vi "Tag Names.vi"(11 "State in":T2={"State"=enum."Idle", "Start Time"=timestamp(0 s since 1904-01-01), "Configuration"={"Cycle Period"=0.0, "Ismatech"={"VISA resource name"="", "Simulated?"=FALSE, "Pump Number"=1.0, "Reverse?"=FALSE}, "Masterflex"={"VISA resource name"="", "Simulated?"=FALSE, "Pump Number"=1.0, "Reverse?"=FALSE}, "Mettler"={"VISA resource name"="", "Simulated?"=FALSE}, "Bronkhorst M13 Flow Meter"={"VISA resource name"="", "Simulated?"=FALSE}, "PID 2 Parameters"={"Input Device"=enum."Bronkhorst M13", "Output Device"=enum."Ismatec ISM 831C", "Setpoint"=0.0, "PID gains"={"proportional gain (Kc)"=1.0, "integral time (Ti, min)"=0.01, "derivative time (Td, min)"=0.0}}, "Manual Entry"=0.0, "Auto?"=TRUE, "output range"={"output high"=100.0, "output low"=0.0}, "Bronkhorst M14"={"VISA resource name"="", "Simulated?"=FALSE}, "Tacmina Settings"={"Analog DAQ Task"="", "Digital DAQ Task"=""}, "KNF SIMDOS Settings"={"VISA resource name"="", "Simulated?"=TRUE}, "ASIA Pump C"={"ASIA Pump #"=0, "channel"=0, "Simulated"=FALSE}, "VICI Settings"={"VISA resource name"="", "Simulated?"=FALSE, "Pump Letter"="", "Reverse?"=FALSE}, "FLOM Settings"={"VISA resource name"="", "Simulated?"=TRUE, "Pump Number"=0.0}, "SSI PR Settings"={"VISA resource name"="", "Simulated?"=FALSE}}, "Current Time"=timestamp(0 s since 1904-01-01), "PID 1 Parameters"={"Setpoint"=0.0, "PID gains"={"proportional gain (Kc)"=1.0, "integral time (Ti, min)"=0.01, "derivative time (Td, min)"=0.0}}, "First Iteration"=FALSE, "Data"={"Flowmeter Output"=0.0, "Density"=0.0, "FL Temp"=0.0, "Scale Output (g)"=0.0, "Scale Rate of Change (g/min)"=0.0, "PID 1 Output"=0.0, "PID 2 Process Variable"=0.0, "PID 2 output"=0.0, "Pump Flow"=0.0, "Pump Pressure"=0.0}, "Process Name"="", "Pump On?"=enum."Off", "Input Error"=FALSE, "Output Error"=FALSE, "Log Started"=FALSE, "Current Setpoint"=0.0} {"PID 1 Parameters"."PID gains"."derivative time (Td, min)" format="%.3f"; "PID 1 Parameters"."PID gains"."integral time (Ti, min)" format="%.3f"; "PID 1 Parameters"."PID gains"."proportional gain (Kc)" format="%.3f"; "Configuration"."output range"."output low" min=0.0 max=100.0 format="%.2f"; "Configuration"."output range"."output high" format="%.2f"; "Configuration"."PID 2 Parameters"."PID gains"."derivative time (Td, min)" format="%.3f"; "Configuration"."PID 2 Parameters"."PID gains"."integral time (Ti, min)" format="%.3f"; "Configuration"."PID 2 Parameters"."PID gains"."proportional gain (Kc)" format="%.3f"; "Configuration"."ASIA Pump C"."channel" min=0 max=1 step=1; "Configuration"."Ismatech"."Pump Number" min=1.0 max=20.0 step=1.0; "Configuration"."Masterflex"."Pump Number" min=1.0 max=20.0 step=1.0}) -> (0 "All  Flow Meter Tags":string[](array[string]), 1 "All  Scale Tags":string[](array[string]), 3 "Feed Module Tag Names":T1, 4 "All Boolean Tags":string[](array[string]), 5 "All  Numeric Tags":string[](array[string]))   [LabVIEW 2018, in "Feed Module.lvlib" / "Feed Module Engine.lvlib"]
uses:
  Feed Module Engine.lvlib
  State Cluster.ctl
  State Enum.ctl
  Feed Module/Controls/Feed Module Settings Cluster.ctl
  Ismatec ISM 831C/Controls/Ismatech Settings Cluster.ctl
  Masterflex 7550-30/Controls/Settings Cluster.ctl
  Mettler Toledo/Controls/Settings Cluster.ctl
  Bronkhorst M13 Flow Meter/Settings Cluster.ctl
  PID 2 Parameters Cluster.ctl
  PID Input Enum.ctl
  PID 2 Output Enum.ctl
  Tacmina QI/Tacmina QI DAQ Setting.ctl
  KNF Pump/Settings Cluster plus SIMDOS.ctl
  ASIA Pump/Pump Settings.ctl
  VICI M50 Party Mode/Settings Cluster.ctl
  FLOM Pump/Settings Cluster.ctl
  SSI PR Class/SSI PR Settings Cluster.ctl
  PID 1 Parameters Cluster.ctl
  Feed Module/Controls/Feed Module Tag Names Cluster.ctl
  Feed Module/Feed Module.lvlib
  Ismatec ISM 831C/Ismatec ISM 831C.lvlib
  Masterflex 7550-30/Masterflex 7550-30.lvlib
  Mettler Toledo/Mettler Toledo.lvlib
  Bronkhorst M13 Flow Meter/Bronkhorst M13 Flow Meter.lvlib
  Tacmina QI/Tacmina QI.lvlib
  KNF Pump/KNF SIMDOS.lvlib
  ASIA Pump.lvlib
  VICI M50 Party Mode/VICI M6 M50 Party Mode.lvlib
  FLOM Pump/FLOM Pump.lvlib
  SSI PR Class/SSI PR Pump.lvlib
panel:
  out "Pump Flow Tag":string
  out "PID 2 Out Tag":string
  out "Scale Tag":string
  # "Output Instruments"
  # "Input Instruments"
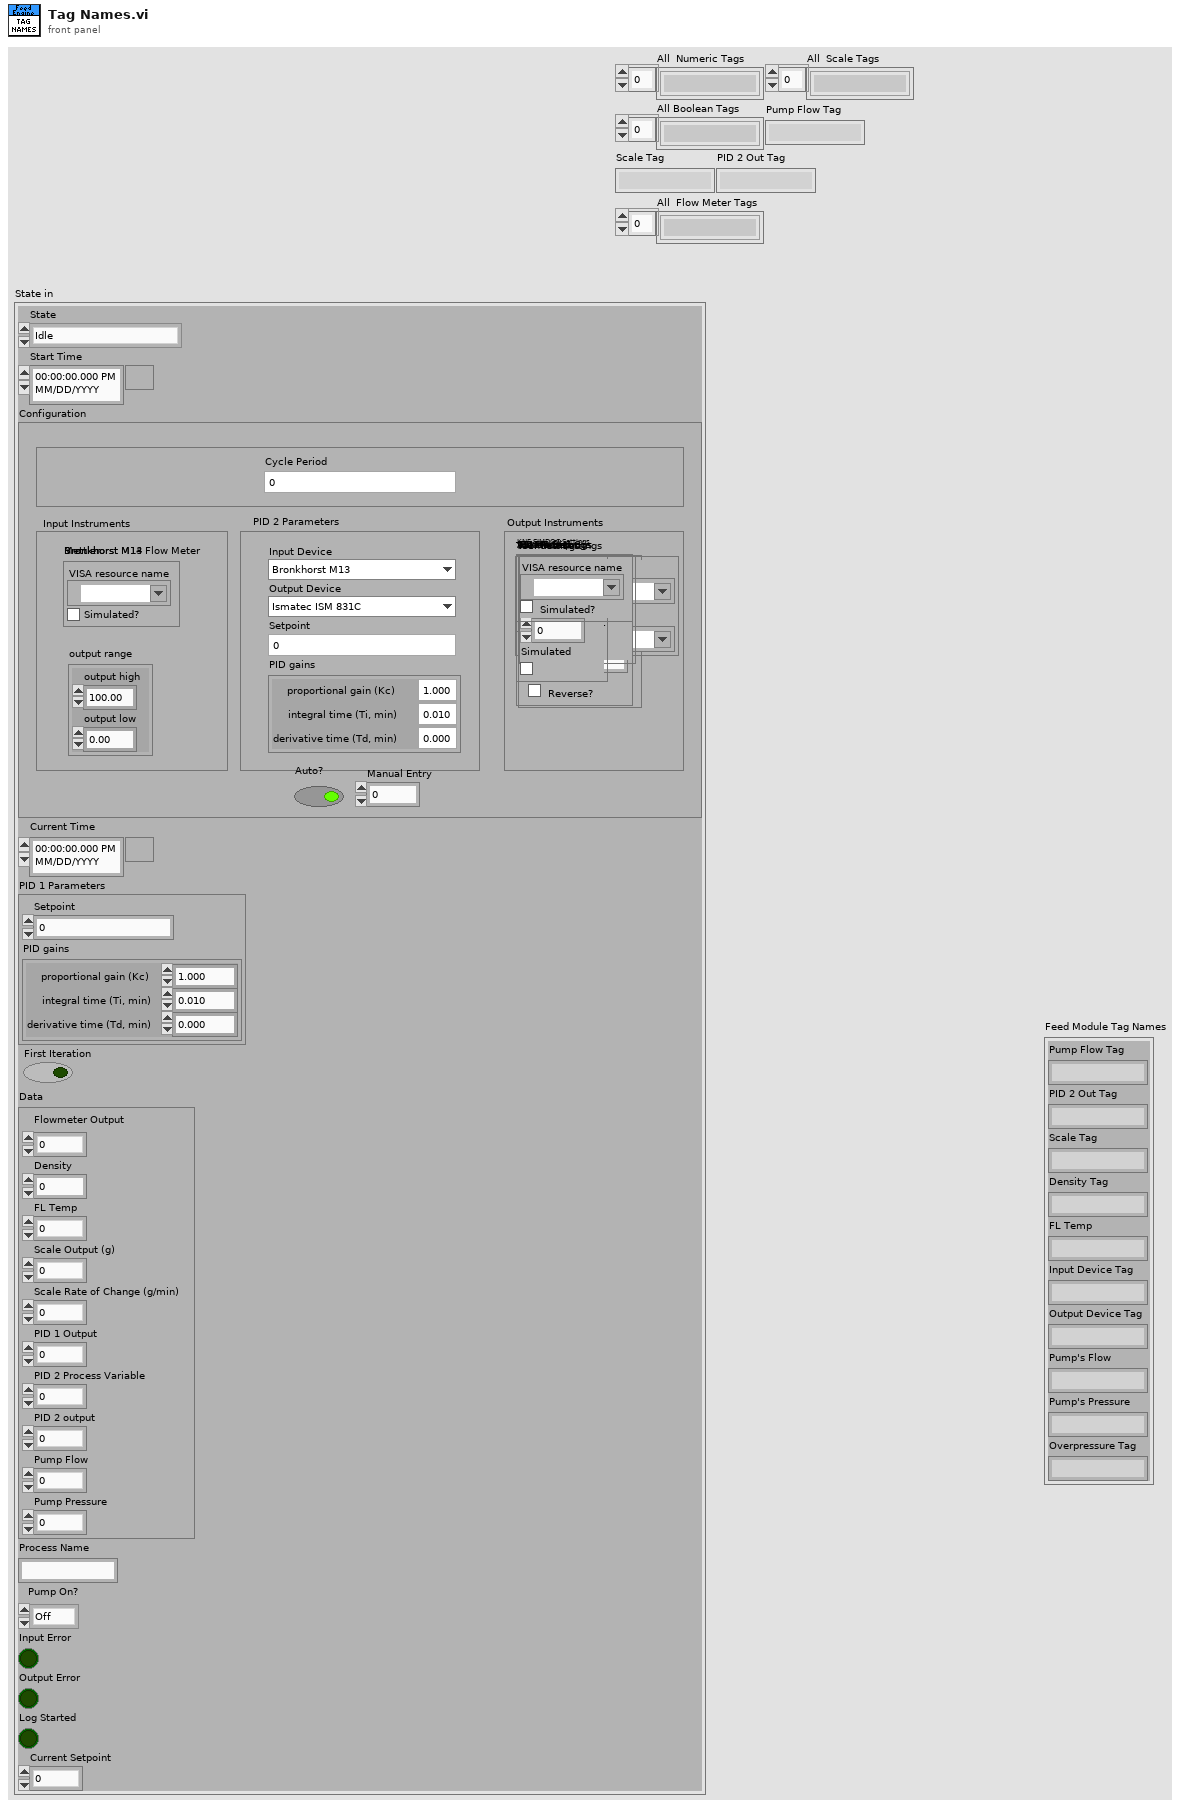
[diagram p1: front panel]
types:
  T1 = typedef "Feed Module.lvlib/Feed Module Tag Names Cluster.ctl" = cluster{"Pump Flow Tag":string, "PID 2 Out Tag":string, "Scale Tag":string, "Density Tag":string, "FL Temp":string, "Input Device Tag":string, "Output Device Tag":string, "Pump's Flow":string, "Pump's Pressure":string, "Overpressure Tag":string}
  T2 = typedef "Feed Module.lvlib/Feed Module Engine.lvlib/State Cluster.ctl" = cluster{"State":T3, "Start Time":timestamp, "Configuration":T4, "Current Time":timestamp, "PID 1 Parameters":T18, "First Iteration":bool, "Data":cluster{"Flowmeter Output":dbl, "Density":dbl, "FL Temp":dbl, "Scale Output (g)":dbl, "Scale Rate of Change (g/min)":dbl, "PID 1 Output":dbl, "PID 2 Process Variable":dbl, "PID 2 output":dbl, "Pump Flow":dbl, "Pump Pressure":dbl}, "Process Name":string, "Pump On?":enum16{"Off", "On", "Not Initialized"}, "Input Error":bool, "Output Error":bool, "Log Started":bool, "Current Setpoint":dbl}
  T3 = typedef "Feed Module.lvlib/Feed Module Engine.lvlib/State Enum.ctl" = enum16{"Measuring", "Idle", "Paused"}
  T4 = typedef "Feed Module.lvlib/Feed Module Settings Cluster.ctl" = cluster{"Cycle Period":dbl, "Ismatech":T5, "Masterflex":T6, "Mettler":T7, "Bronkhorst M13 Flow Meter":T8, "PID 2 Parameters":T9, "Manual Entry":dbl, "Auto?":bool, "output range":cluster{"output high":dbl, "output low":dbl}, "Bronkhorst M14":T7, "Tacmina Settings":T12, "KNF SIMDOS Settings":T13, "ASIA Pump C":T14, "VICI Settings":T15, "FLOM Settings":T16, "SSI PR Settings":T17}
  T5 = typedef "Ismatec ISM 831C.lvlib/Ismatech Settings Cluster.ctl" = cluster{"VISA resource name":refnum<visa-resource-name>, "Simulated?":bool, "Pump Number":dbl, "Reverse?":bool}
  T6 = typedef "Masterflex 7550-30.lvlib/Settings Cluster.ctl" = cluster{"VISA resource name":refnum<visa-resource-name>, "Simulated?":bool, "Pump Number":dbl, "Reverse?":bool}
  T7 = typedef "Mettler Toledo.lvlib/Settings Cluster.ctl" = cluster{"VISA resource name":refnum<visa-resource-name>, "Simulated?":bool}
  T8 = typedef "Bronkhorst M13 Flow Meter.lvlib/Settings Cluster.ctl" = cluster{"VISA resource name":refnum<visa-resource-name>, "Simulated?":bool}
  T9 = typedef "PID 2 Parameters Cluster.ctl" = cluster{"Input Device":T10, "Output Device":T11, "Setpoint":dbl, "PID gains":cluster{"proportional gain (Kc)":dbl, "integral time (Ti, min)":dbl, "derivative time (Td, min)":dbl}}
  T10 = typedef "PID Input Enum.ctl" = enum16{"Default", "Bronkhorst M13", "Bronkhorst M14", "Scale Rate of Change"}
  T11 = typedef "PID 2 Output Enum.ctl" = enum16{"Default", "Ismatec ISM 831C", "Masterflex 7550-30", "VICI", "Tacmina QI", "KNF SIMDOS", "ASIA Type C", "FLOM UI-22-11", "SSI PR"}
  T12 = typedef "Tacmina QI.lvlib/Tacmina QI DAQ Setting.ctl" = cluster{"Analog DAQ Task":refnum<k21>, "Digital DAQ Task":refnum<k21>}
  T13 = typedef "KNF SIMDOS.lvlib/Settings Cluster plus SIMDOS.ctl" = cluster{"VISA resource name":refnum<visa-resource-name>, "Simulated?":bool}
  T14 = typedef "ASIA Pump.lvlib/Pump Settings.ctl" = cluster{"ASIA Pump #":i32, "channel":i32, "Simulated":bool}
  T15 = typedef "VICI M6 M50 Party Mode.lvlib/Settings Cluster.ctl" = cluster{"VISA resource name":refnum<visa-resource-name>, "Simulated?":bool, "Pump Letter":string, "Reverse?":bool}
  T16 = typedef "FLOM Pump.lvlib/Settings Cluster.ctl" = cluster{"VISA resource name":refnum<visa-resource-name>, "Simulated?":bool, "Pump Number":dbl}
  T17 = typedef "SSI PR Pump.lvlib/SSI PR Settings Cluster.ctl" = cluster{"VISA resource name":refnum<visa-resource-name>, "Simulated?":bool}
  T18 = typedef "PID 1 Parameters Cluster.ctl" = cluster{"Setpoint":dbl, "PID gains":cluster{"proportional gain (Kc)":dbl, "integral time (Ti, min)":dbl, "derivative time (Td, min)":dbl}}
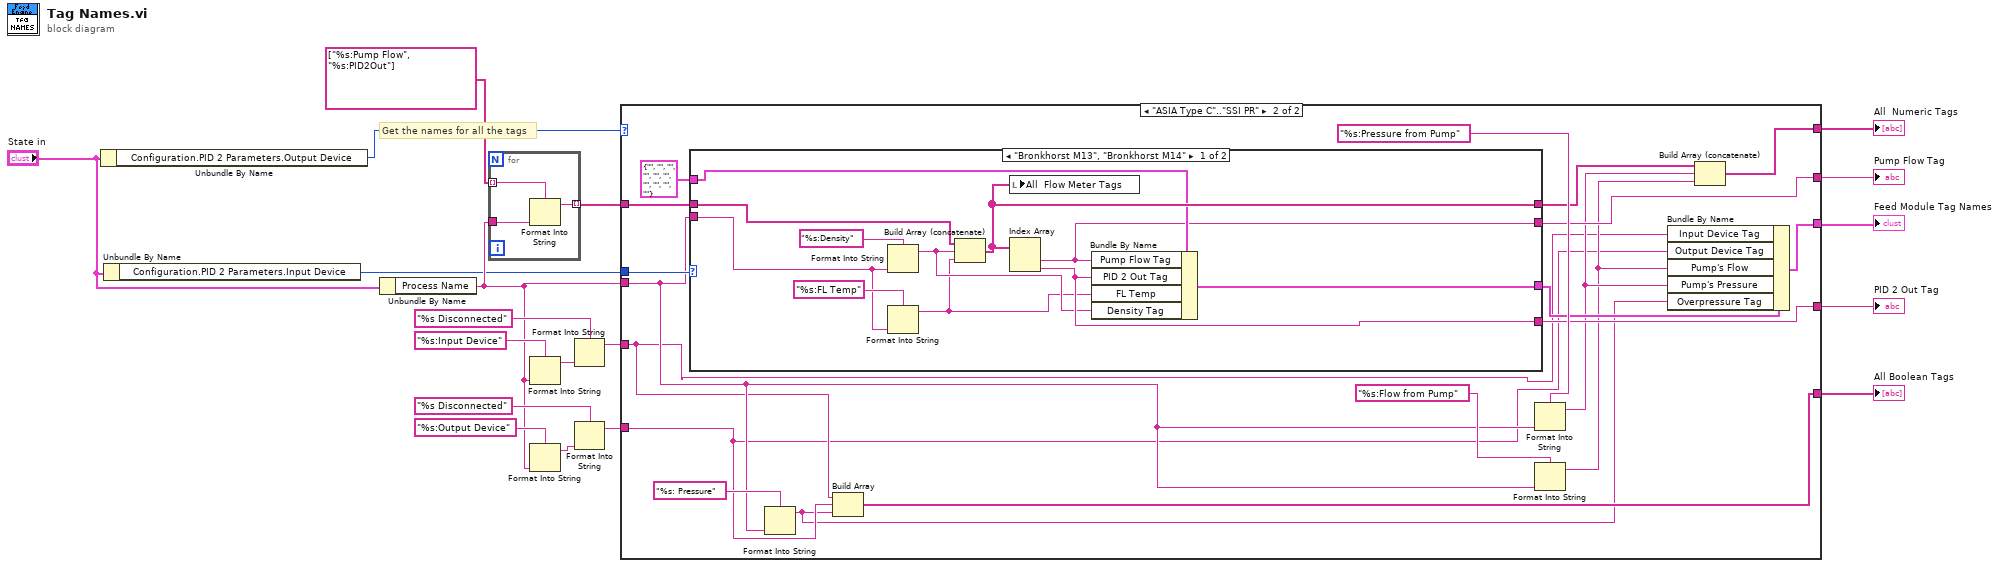
[diagram p0: block diagram]
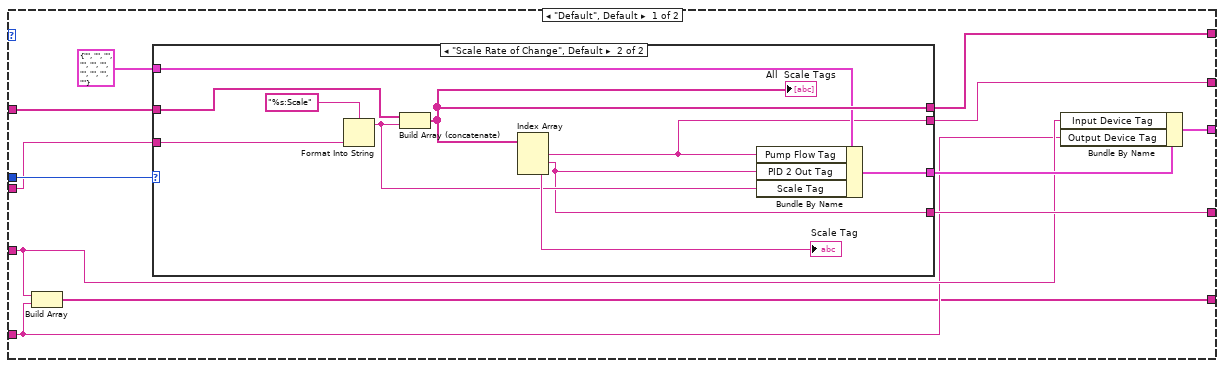
[diagram p2: hidden frame]
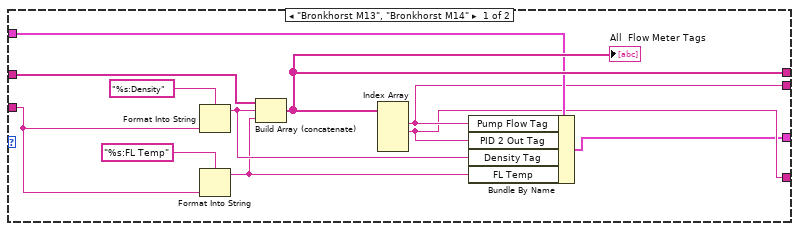
[diagram p3: hidden frame]
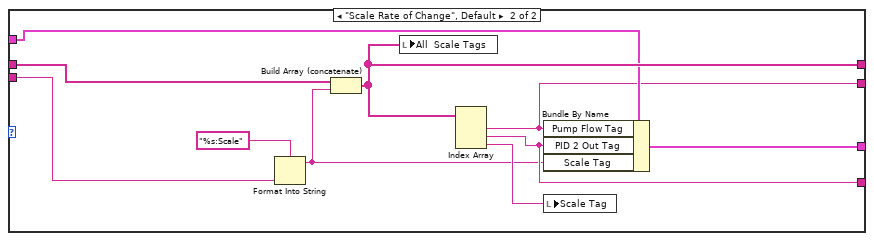
[diagram p4: hidden frame]
diagram:
  # "Get the names for all the tags"
  n1 = Unbundle By Name("State in") -> ("Configuration.PID 2 Parameters.Output Device"=w12:T11)
  n2 = Unbundle By Name("State in") -> ("Configuration.PID 2 Parameters.Input Device"=w10:T10)
  n3 = Unbundle By Name("State in") -> ("Process Name"=w11:string)
  n4 = for {
    tunnel: string[] ["%s:Pump Flow", "%s:PID2Out"] -> [w22] mode=indexing
    tunnel: w11 -> [w21]
    tunnel: [w20] -> w9 mode=indexing
    n5 = Format Into String(format string=w22, w21) -> (resulting string=w20:string)  [unwired: 2 in, 1 out]
  }
  n6 = Format Into String(format string="%s:Input Device", w11) -> (resulting string=w16:string)  [unwired: 2 in, 1 out]
  n7 = Format Into String(format string="%s:Output Device", w11) -> (resulting string=w15:string)  [unwired: 2 in, 1 out]
  n8 = Format Into String(format string="%s Disconnected", w16) -> (resulting string=w3:string)  [unwired: 2 in, 1 out]
  n9 = Format Into String(format string="%s Disconnected", w15) -> (resulting string=w2:string)  [unwired: 2 in, 1 out]
  n10 = case shown="\"ASIA Type C\"..\"SSI PR\"" w12 {
    tunnel: w11 -> [w32 w60]
    tunnel: w10 -> [w34 w72]
    tunnel: w9 -> [w33 w71]
    tunnel: [w31 w70] -> w8
    tunnel: [w30 w68] -> w5
    tunnel: [w29 w67] -> w6
    tunnel: [w28 w64] -> w4
    tunnel: w3 -> [w25 w59]
    tunnel: w2 -> [w24 w58]
    tunnel: [w23 w57] -> w1
    frame "Default", Default {
      n11 = Build Array(w25, w24) -> (w23:string[])
      n12 = case shown="\"Scale Rate of Change\", Default" w34 {
        tunnel: w33 -> [w43 w55]
        tunnel: [w41 w52] -> w31
        tunnel: w32 -> [w42 w53]
        tunnel: [w39 w48] -> w29
        tunnel: [w38 w46] -> w30
        tunnel: T1 {"Pump Flow Tag"="", "PID 2 Out Tag"="", "Scale Tag"="", "Density Tag"="", "FL Temp"="", "Input Device Tag"="", "Output Device Tag"="", "Pump's Flow"="", "Pump's Pressure"="", "Overpressure Tag"=""} ("Feed Module Tag Names") -> [w40 w50]
        tunnel: [w37 w49] -> w26
        frame "Bronkhorst M13", "Bronkhorst M14" {
          n13 = Format Into String(format string="%s:Density", w42) -> (resulting string=w36:string)  [unwired: 2 in, 1 out]
          n14 = Format Into String(format string="%s:FL Temp", w42) -> (resulting string=w35:string)  [unwired: 2 in, 1 out]
          n15 = Build Array (concatenate)(w43, w36, w35) -> (w41:string[])
          "All  Flow Meter Tags" <- w41
          n16 = Index Array(array=w41) -> (element #1=w39:string, element #2=w38:string)  [unwired: 4 in, 2 out]
          n17 = Bundle By Name(cluster=w40, "Pump Flow Tag"=w39, "PID 2 Out Tag"=w38, "Density Tag"=w36, "FL Temp"=w35) -> (w37:T1)
        }
        frame "Scale Rate of Change", Default {
          n18 = Format Into String(format string="%s:Scale", w53) -> (resulting string=w47:string)  [unwired: 2 in, 1 out]
          n19 = Build Array (concatenate)(w55, w47) -> (w52:string[])
          "All  Scale Tags" <- w52
          n20 = Index Array(array=w52) -> (element #1=w48:string, element #2=w46:string, element #3=→"Scale Tag":string)  [unwired: 3 in]
          n21 = Bundle By Name(cluster=w50, "Pump Flow Tag"=w48, "PID 2 Out Tag"=w46, "Scale Tag"=w47) -> (w49:T1)
        }
      }
      n22 = Bundle By Name(cluster=w26, "Input Device Tag"=w25, "Output Device Tag"=w24) -> (w28:T1)
    }
    frame "ASIA Type C".."SSI PR" {
      n23 = case shown="\"Bronkhorst M13\", \"Bronkhorst M14\"" w72 {
        tunnel: w71 -> [w83 w95]
        tunnel: [w81 w92] -> w69
        tunnel: w60 -> [w82 w93]
        tunnel: [w79 w87] -> w67
        tunnel: [w78 w88] -> w68
        tunnel: T1 {"Pump Flow Tag"="", "PID 2 Out Tag"="", "Scale Tag"="", "Density Tag"="", "FL Temp"="", "Input Device Tag"="", "Output Device Tag"="", "Pump's Flow"="", "Pump's Pressure"="", "Overpressure Tag"=""} ("Feed Module Tag Names") -> [w80 w91]
        tunnel: [w77 w90] -> w65
        frame "Bronkhorst M13", "Bronkhorst M14" {
          n24 = Format Into String(format string="%s:Density", w82) -> (resulting string=w76:string)  [unwired: 2 in, 1 out]
          n25 = Format Into String(format string="%s:FL Temp", w82) -> (resulting string=w75:string)  [unwired: 2 in, 1 out]
          n26 = Build Array (concatenate)(w83, w76, w75) -> (w81:string[])
          n27 = local write "All  Flow Meter Tags"(w81) -> ()
          n28 = Index Array(array=w81) -> (element #1=w79:string, element #2=w78:string)  [unwired: 2 in]
          n29 = Bundle By Name(cluster=w80, "Pump Flow Tag"=w79, "PID 2 Out Tag"=w78, "FL Temp"=w75, "Density Tag"=w76) -> (w77:T1)
        }
        frame "Scale Rate of Change", Default {
          n30 = Format Into String(format string="%s:Scale", w93) -> (resulting string=w86:string)  [unwired: 2 in, 1 out]
          n31 = Build Array (concatenate)(w95, w86) -> (w92:string[])
          n32 = local write "All  Scale Tags"(w92) -> ()
          n33 = Index Array(array=w92) -> (element #1=w87:string, element #2=w88:string, element #3=w89:string)  [unwired: 3 in]
          n34 = Bundle By Name(cluster=w91, "Pump Flow Tag"=w87, "PID 2 Out Tag"=w88, "Scale Tag"=w86) -> (w90:T1)
          n35 = local write "Scale Tag"(w89) -> ()
        }
      }
      n36 = Format Into String(format string="%s: Pressure", w60) -> (resulting string=w56:string)  [unwired: 2 in, 1 out]
      n37 = Build Array(w59, w58, w56) -> (w57:string[])
      n38 = Format Into String(format string="%s:Pressure from Pump", w60) -> (resulting string=w63:string)  [unwired: 2 in, 1 out]
      n39 = Format Into String(format string="%s:Flow from Pump", w60) -> (resulting string=w62:string)  [unwired: 2 in, 1 out]
      n40 = Bundle By Name(cluster=w65, "Input Device Tag"=w59, "Output Device Tag"=w58, "Pump's Flow"=w62, "Pump's Pressure"=w63, "Overpressure Tag"=w56) -> (w64:T1)
      n41 = Build Array (concatenate)(w69, w63, w62) -> (w70:string[])
    }
  }
  "All  Numeric Tags" <- w8
  "All Boolean Tags" <- w1
  "PID 2 Out Tag" <- w5
  "Pump Flow Tag" <- w6
  "Feed Module Tag Names" <- w4
